vi "Capture timing.vi"() -> ()   [LabVIEW 2018]
doc: "The intent for this application is to demonstrate the performance of the different Windows 10 priority settings"
uses:
  application-priority/Priority Levels..enum.ctl
  <vilib>/Platform/TimedLoop/XDataNode/timing_clust.ctl
  <vilib>/Platform/TimedLoop/XDataNode/nitl_modes.ctl
  <vilib>/Platform/TimedLoop/XDataNode/wakeup.ctl
  <vilib>/platform/TimedLoop/XDataNode/XDataNode.xnode
  <vilib>/Platform/TimedLoop/XDataNode/XDNodeRunTimeDep.lvlib
panel:
  in  "Result Folder path":path=path "D:/Priority Benchmarking/Results"
  out "p":string
  in  "Piority":T1[](array[typedef])
  out "i1":i32
  in  "Number of loops":i32[](array[numeric])
  in  "Period (ms)":i64=5
  out "i2":i32
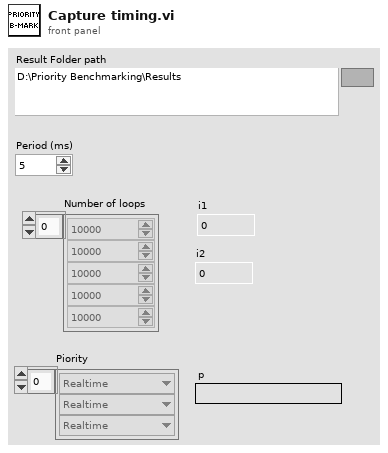
[diagram p1: front panel]
types:
  T1 = typedef "Priority Levels..enum.ctl" = enum16{"Realtime", "High", "Above normal", "Normal", "Below normal", "Low"}
  T2 = enum16{"open", "open or create", "create or replace", "create", "open (read-only)"}
  T3 = typedef "XDNodeRunTimeDep.lvlib/timing_clust.ctl" = cluster{"Expected End [f-1]":u64, "Actual End [f-1]":u64, "Finished Late? [f-1]":bool, "Expected End [i-1]":u64, "Actual End [i-1]":u64, "Finished Late? [i-1]":bool, "Expected Start [i]":u64, "Actual Start [i]":u64, "Expected Start [f]":u64, "Actual Start [f]":u64, "Source Name":string, "Structure Name":string, "Period":i64, "Deadline":i64, "Offset":i64, "Start":i64, "Priority":i32, "Timeout":i32, "Mode":T4, "Wakeup Reason":T5, "Error":errorcluster, "Source Type":string, "Secondary Source Type":string, "Global End Time":u64, "Global Start Time":u64, "Frame Duration":u64, "Iteration Duration":u64, "Assigned CPU":i32, "I/O Scan Engine Mode":u32}
  T4 = typedef "XDNodeRunTimeDep.lvlib/nitl_modes.ctl" = enum32{"No Change", "Process missed periods, maintain original phase", "Discard missed periods, maintain original phase", "Process missed periods, ignore original phase", "Discard missed periods, ignore original phase"}
  T5 = typedef "XDNodeRunTimeDep.lvlib/wakeup.ctl" = enum32{"Normal", "Aborted", "Asynchronous wakeup", "Timing source error", "Timed loop error", "Timeout"}
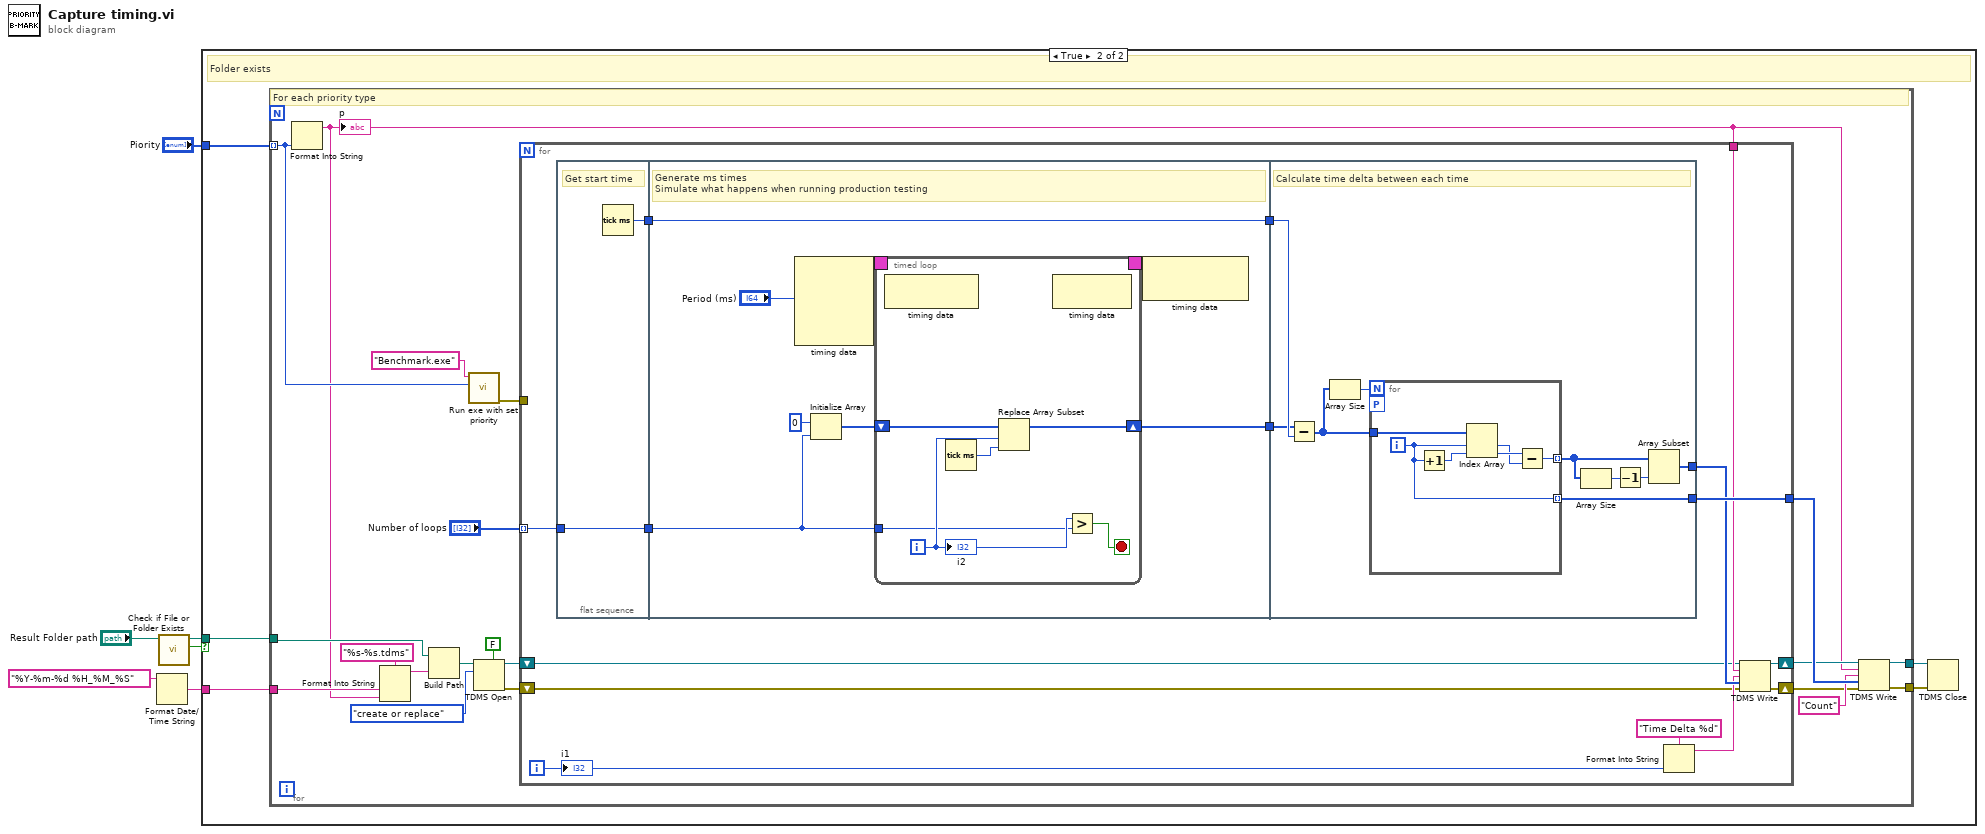
[diagram p0: block diagram]
diagram:
  n1 = Format Date/Time String(time format string (%c)="%Y-%m-%d %H_%M_%S") -> (date/time string=w4:string)  [unwired: 2 out]
  n2 = call <vilib>:"Check if File or Folder Exists.vi"("path"="Result Folder path") -> ("file or folder exists?"=w1:bool, "dup path"=w2:path)  [unwired: 8 in, 1 out]
  n3 = case shown="True" w1 {
    tunnel: "Piority" -> [_ w11]
    tunnel: w4 -> [_ w8]
    tunnel: w2 -> [_ w7]
    frame False {
    }
    frame True {
      # "Folder exists"
      n4 = for {
        tunnel: w11 -> [w29] mode=indexing
        tunnel: [w23] -> w10
        tunnel: [w24] -> w9
        tunnel: w8 -> [w18]
        tunnel: w7 -> [w17]
        # "For each priority type"
        n5 = Format Into String(w29) -> (resulting string=w12:string)  [unwired: 3 in, 1 out]
        "p" <- w12
        n6 = Format Into String(format string="%s-%s.tdms", w18, w12) -> (resulting string=w21:string)  [unwired: 2 in, 1 out]
        n7 = Build Path(base path=w17, name or relative path=w21) -> (appended path=w20:path)
        n8 = call "Run exe with set priority.vi"("Priority Levels (Normal)"=w29, "Process name (abc.exe)"="Benchmark.exe") -> ("error out"=w30:errorcluster)  [unwired: 9 in]
        n9 = TDMS Open(5:FALSE ("create index file? (T)"), 10:T2."create or replace" ("operation (0:open)"), 11:w20) -> (0:w13:errorcluster, 3:w14:refnum<k34>)  [unwired: 4 in]
        n10 = for {
          tunnel: "Number of loops" -> [w42] mode=indexing
          tunnel: w30 -> [_]
          tunnel: [w41] -> w28
          tunnel: w12 -> [w37]
          shift-right: [w35] -> w22
          shift-left: w14 -> [w33]
          shift-right: [w34] -> w25
          shift-left: w13 -> [w32]
          i -> [w39]
          n11 = flat-sequence {
            tunnel: w42 -> [w48]
            tunnel: [w48] -> w44
            tunnel: [w47] -> w43
            tunnel: [w53] -> w46
            tunnel: [w50] -> w45
            tunnel: w44 -> [w49]
            tunnel: w43 -> [w53]
            tunnel: [w77] -> w38
            tunnel: w46 -> [w76]
            tunnel: w45 -> [w75]
            tunnel: [w69] -> w41
            frame #0 {
              # "Get start time"
              n12 = Tick Count (ms)() -> (millisecond timer value=w47:u32)
            }
            frame #1 {
              # "Generate ms times\nSimulate what happens when running production testing"
              n13 = node-c288("Period (ms)") -> (w56:T3)  [unwired: 3 in]
              n14 = Initialize Array(u32 0 ("element"), w49) -> (w51:u32[])
              n15 = timed-loop {
                timing: w56 -> [_]
                timing-out: [_] -> w55
                shift-right: [w60] -> w50
                shift-left: w51 -> [w61]
                tunnel: w49 -> [w57]
                i -> [w59]
                stop <- w62 stop-if-true
                n16 = node-c288() -> ()  [unwired: 1 in, 1 out]
                n17 = Tick Count (ms)() -> (millisecond timer value=w58:u32)
                n18 = Replace Array Subset(array=w61, new element=w58, index=w59) -> (w60:u32[])
                n19 = node-c288() -> ()  [unwired: 1 in, 1 out]
                n20 = Greater?(x=w59, y=w57) -> (0:w62:bool)
                "i2" <- w59
              }
              n21 = node-c288(w55) -> ()  [unwired: 1 out]
            }
            frame #2 {
              # "Calculate time delta between each time"
              n22 = Subtract(x=w75, y=w76) -> (x-y=w71:u32[])
              n23 = Array Size(array=w71) -> (size(s)=w70:i32)
              n24 = for {
                N: w70 -> [_]
                tunnel: w71 -> [w83]
                tunnel: [w79] -> w73 mode=indexing
                workers-P: _ -> [_]
                tunnel: [w78] -> w69 mode=indexing
                i -> [w78]
                n25 = Increment(x=w78) -> (x+1=w82:i32)
                n26 = Index Array(array=w83, index #1=w78, index #2=w82) -> (element #1=w80:u32, element #2=w81:u32)
                n27 = Subtract(x=w81, y=w80) -> (x-y=w79:u32)
              }
              n28 = Array Size(array=w73) -> (size(s)=w74:i32)
              n29 = Decrement(x=w74) -> (x-1=w72:i32)
              n30 = Array Subset(array=w73, length=w72) -> (w77:u32[])  [unwired: 1 in]
            }
          }
          n31 = Format Into String(format string="Time Delta %d", w39) -> (resulting string=w36:string)  [unwired: 2 in, 1 out]
          n32 = TDMS Write(0:w33, 5:w37, 7:w36, 9:w38, 11:w32) -> (4:w35:refnum<k34>, 15:w34:errorcluster)  [unwired: 1 in, 2 out]
          "i1" <- w39
        }
        n33 = TDMS Write(0:w22, 5:w12, 7:"Count", 9:w28, 11:w25) -> (4:w23:refnum<k34>, 15:w24:errorcluster)  [unwired: 1 in, 2 out]
      }
      n34 = TDMS Close(8:w9, 11:w10) -> ()  [unwired: 2 out]
    }
  }
